vi "Modbus Read STR8.vi"(7 "Slave Address":u8, 8 "error in (no error)":errorcluster, 10 "Register Start Address":u16 format="%x", 11 "VISA resource in":refnum<visa-resource-name>) -> (0 "error out":errorcluster, 1 "Output string (8 chars)":string, 3 "VISA resource out":refnum<visa-resource-name>)   [LabVIEW 2023, in "Voegtlin_NI_SMART_Modbus_Drivers.lvlib"]
doc: "Lese einen String mit 8 Zeichen an der angegebenen Startadresse des selektierten Geraetes aus.\nDer COM-Port muss dazu initialisiert sein (benutze\" Modbus Init.vi\")."
uses:
  Voegtlin_NI_SMART_Modbus_Drivers.lvlib
  Enums/Modbus Comm.ctl
panel:
  out "Outputdata U8 (array)":u8[](array[numeric])
  out "Read register data\n U16 (array)":u16[](array[numeric])
  # "Input Data"
  # "Internal Data"
  # "Output Data"
  # "(Inputmaske in HEX)"
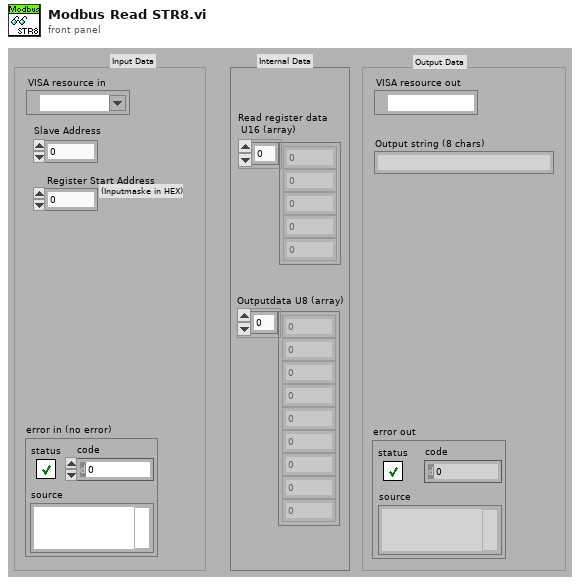
[diagram p1: front panel]
types:
  T1 = typedef "Voegtlin_NI_SMART_Modbus_Drivers.lvlib/Modbus Comm.ctl" = enum16{"Init", "Read", "Write", "Exit"}
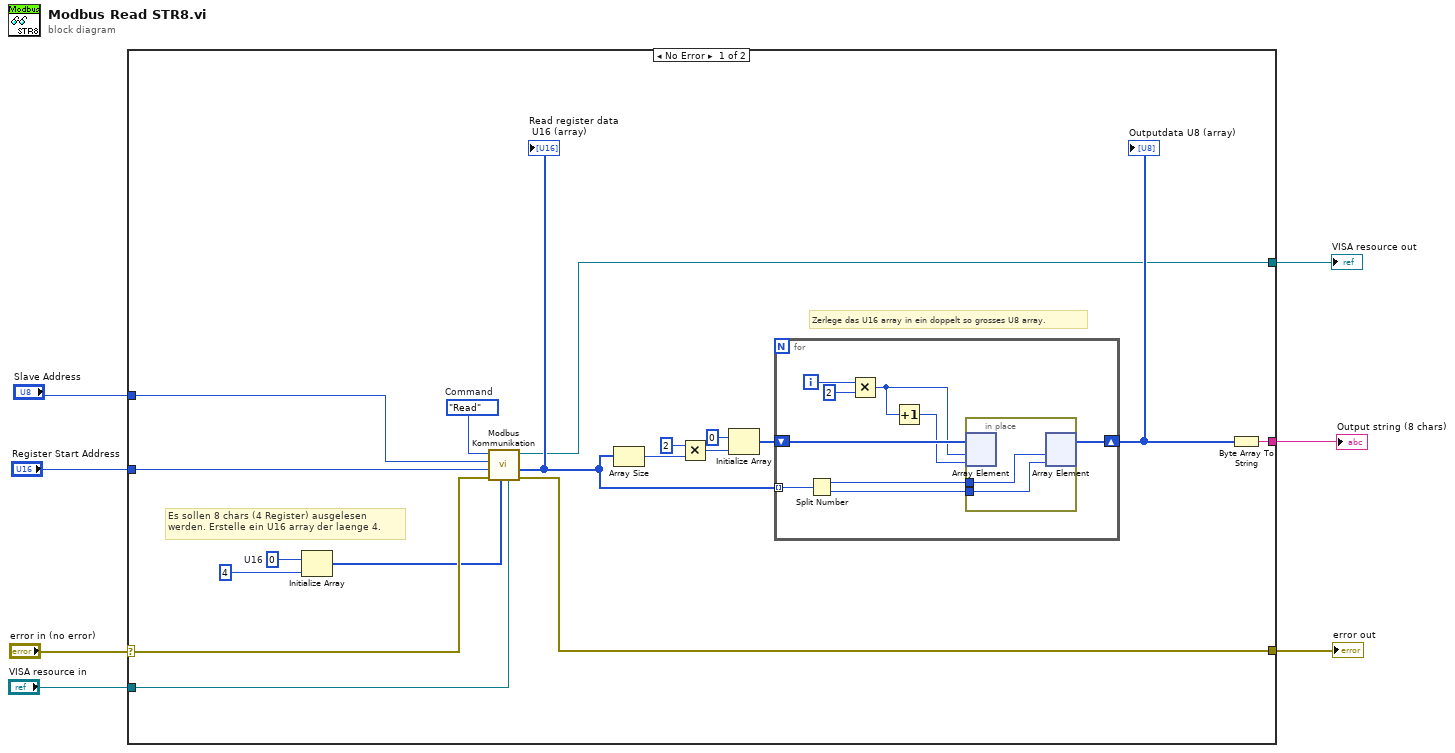
[diagram p0: block diagram]
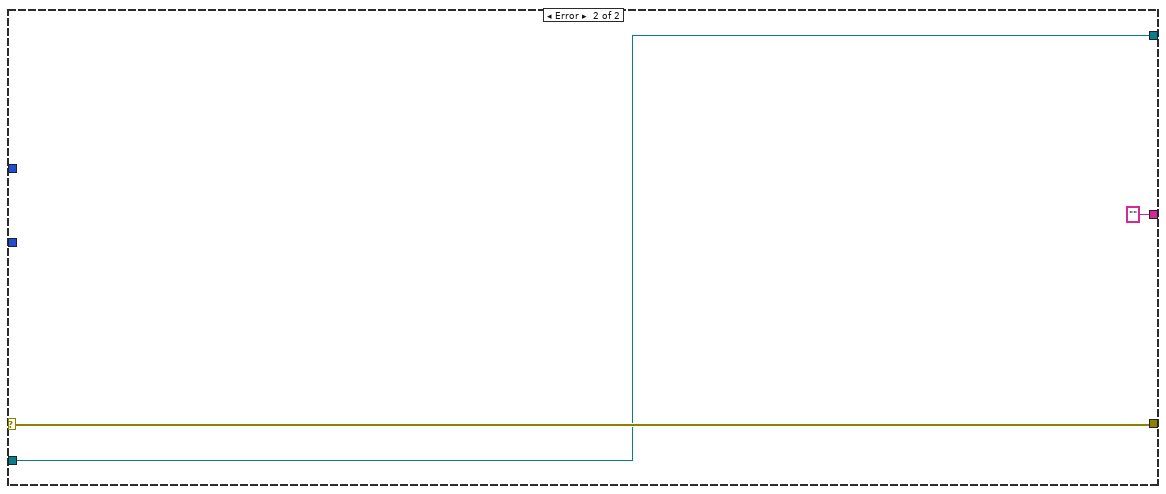
[diagram p2: hidden frame]
diagram:
  n1 = case shown="No Error" "error in (no error)" {
    selector: "error in (no error)" -> [w13 w39]
    tunnel: "Register Start Address" -> [w11 _]
    tunnel: [w25 w39] -> w6
    tunnel: [w16 "" ("string")] -> w5
    tunnel: "Slave Address" -> [w10 _]
    tunnel: "VISA resource in" -> [w9 w37]
    tunnel: [w8 w37] -> w1
    frame No Error {
      w23 = u16 0  # U16
      w24 = Modbus_Comm."Read"  # Command
      # "Zerlege das U16 array in ein doppelt so grosses U8 array."
      # "Es sollen 8 chars (4 Register) ausgelesen werden. Erstelle ein U16 array der laenge 4."
      n2 = Initialize Array(w23, 4) -> (w12:u16[])
      n3 = call "Modbus Kommunikation.vi"("VISA resource in"=w9, "Data In / #Reads [U16]"=w12, "error in (no error)"=w13, "Register Start Address"=w11, "Slave Address"=w10, "Command"=w24) -> ("error out"=w25:errorcluster, "Data Out [U16]"=w17:u16[], "VISA resource out"=w8:refnum<visa-resource-name>)  [unwired: 3 in]
      "Read register data\n U16 (array)" <- w17
      n4 = Array Size(array=w17) -> (size(s)=w22:i32)
      n5 = Multiply(x=2, y=w22) -> (x*y=w20:i32)
      n6 = Initialize Array(u8 0 ("x"), w20) -> (w18:u8[])
      n7 = for {
        tunnel: w17 -> [w34] mode=indexing
        shift-right: [w26] -> w15
        shift-left: w18 -> [w31]
        i -> [w33]
        n8 = Split Number(x=w34) -> (hi(x)=w28:u8, lo(x)=w27:u8)
        n9 = Multiply(x=w33, y=2) -> (x*y=w30:i32)
        n10 = Increment(x=w30) -> (x+1=w29:i32)
        n11 = in-place {
          in-place-border: w28 -> [w36]
          in-place-border: w27 -> [w35]
          n12 = in-place-array #1(w31, w30, w29) -> ()  [unwired: 2 out]
          n13 = in-place-array #1(w36, w35) -> (w26:u8[])  [unwired: 2 out]
        }
      }
      "Outputdata U8 (array)" <- w15
      n14 = Byte Array To String(unsigned byte array=w15) -> (string=w16:string)
    }
    frame Error {
    }
  }
  "error out" <- w6
  "Output string (8 chars)" <- w5
  "VISA resource out" <- w1
